vi "Read Configuration (INI) File.vi"() -> ()   [LabVIEW 2023]
doc: "Illustrates how to read a configuration settings file. Run Write Configuration (INI) File.vi. Then run this VI."
uses:
  <vilib>/Utility/config.llb/Read Key (Boolean).vi
  <vilib>/Utility/config.llb/Read Key (Double).vi
  <vilib>/Utility/config.llb/Read Key (Path).vi
  <vilib>/Utility/config.llb/Read Key (String).vi
  <vilib>/Utility/config.llb/NI_LVConfig.lvlib
panel:
  out "Path Value":path
  out "Numeric Value":dbl
  out "Boolean Value":bool
  out "String 2 Value":string
  out "String 1 Value":string
  # "Overview: Demonstrates the use of the Configuration File VIs to read data from a configuration (INI) file.\nInstructions:\n1. Make sure you have already run Write Configuration (INI) File.vi.\n2. Run this VI. The contents of the configuration file will be displayed below.\n3. Delete the INI file (located at [LabVIEW Data]\\Example Configuration File.ini) when you are done."
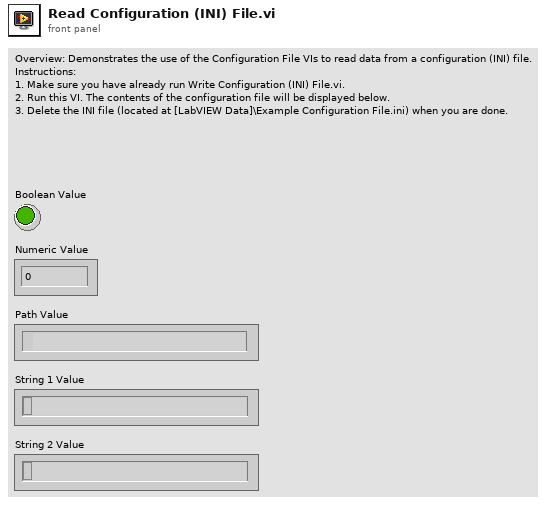
[diagram p1: front panel]
types:
  T1 = typedef "NI_LVConfig.lvlib/Config Data RefNum.ctl" = refnum<k1>
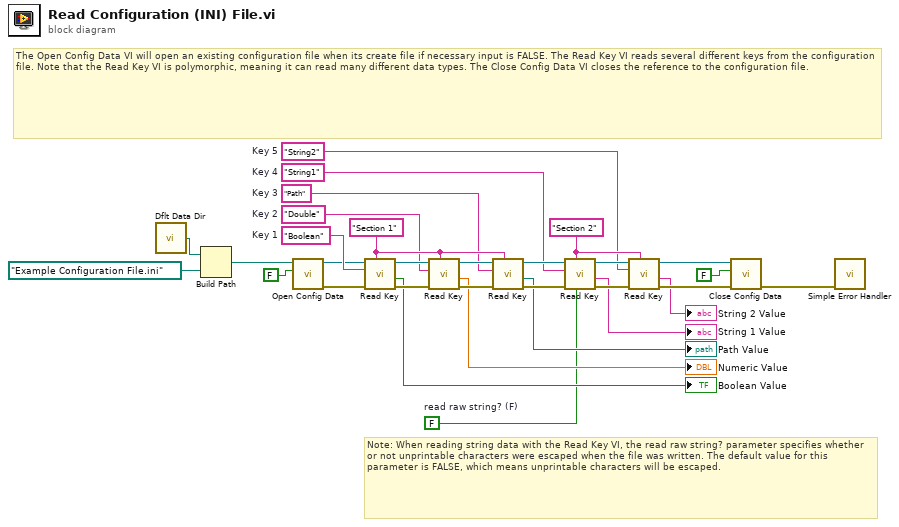
[diagram p0: block diagram]
diagram:
  w5 = FALSE  # read raw string? (F)
  w15 = "String2"  # Key 5
  w16 = "String1"  # Key 4
  w17 = "Path"  # Key 3
  w18 = "Double"  # Key 2
  w19 = "Boolean"  # Key 1
  w20 = "Section 2" ("section")
  w21 = "Section 1" ("section")
  # "The Open Config Data VI will open an existing configuration file when its create file if necessary input is FALSE. The Read Key VI reads several different keys from the configuration file. Note that the Read Key VI is polymorphic, meaning it can read many different data types. The Close Config Data VI closes the reference to the configuration file."
  # "Note: When reading string data with the Read Key VI, the read raw string? parameter specifies whether or not unprintable characters were escaped when the file was written. The default value for this parameter is FALSE, which means unprintable characters will be escaped."
  n1 = call <vilib>:"Dflt Data Dir.vi"() -> ("App:Default Data Directory"=w3:path)
  n2 = Build Path(base path=w3, name or relative path=path "Example Configuration File.ini" ("default name")) -> (appended path=w1:path)
  n3 = call <vilib>:"Open Config Data.vi"("create file if necessary (T)"=FALSE ("create file if necessary? (T)"), "configuration file path"=w1) -> ("error out"=w14:errorcluster, "refnum"=w13:T1)  [unwired: 7 in, 1 out]
  n4 = call-poly <vilib>:"Read Key.vi"("section"=w21, "error in (no error)"=w14, "key"=w19, "refnum"=w13) -> ("error out"=w31:errorcluster, "value"=→"Boolean Value":bool, "refnum out"=w29:T1)  [unwired: 1 in, 4 out]
  n5 = call-poly <vilib>:"Read Key.vi"("section"=w21, "error in (no error)"=w31, "key"=w18, "refnum"=w29) -> ("error out"=w26:errorcluster, "value"=→"Numeric Value":dbl, "refnum out"=w27:T1)  [unwired: 1 in, 4 out]
  n6 = call-poly <vilib>:"Read Key.vi"("section"=w21, "error in (no error)"=w26, "key"=w17, "refnum"=w27) -> ("error out"=w30:errorcluster, "value"=→"Path Value":path, "refnum out"=w28:T1)  [unwired: 1 in, 4 out]
  n7 = call-poly <vilib>:"Read Key.vi"("read raw string? (F)"=w5, "section"=w20, "error in (no error)"=w30, "key"=w16, "refnum"=w28) -> ("error out"=w23:errorcluster, "value"=→"String 1 Value":string, "refnum out"=w22:T1)  [unwired: 1 in, 3 out]
  n8 = call-poly <vilib>:"Read Key.vi"("section"=w20, "error in (no error)"=w23, "key"=w15, "refnum"=w22) -> ("error out"=w25:errorcluster, "value"=→"String 2 Value":string, "refnum out"=w24:T1)  [unwired: 2 in, 3 out]
  n9 = call <vilib>:"Close Config Data.vi"("error in (no error)"=w25, "write file if changed (T)"=FALSE ("write configuration file? (T)"), "refnum"=w24) -> ("error out"=w4:errorcluster)  [unwired: 8 out]
  n10 = call <vilib>:"Simple Error Handler.vi"("error in (no error)"=w4) -> ()  [unwired: 1 in, 8 out]
